vi "ConvertPath.vi"(8 "error in (no error)":errorcluster caption="错误输入（无错误）", 11 "输入路径":path) -> (0 "error out":errorcluster caption="错误输出", 2 "转换后路径":path, 3 "转换前路径":path)   [LabVIEW 2018]
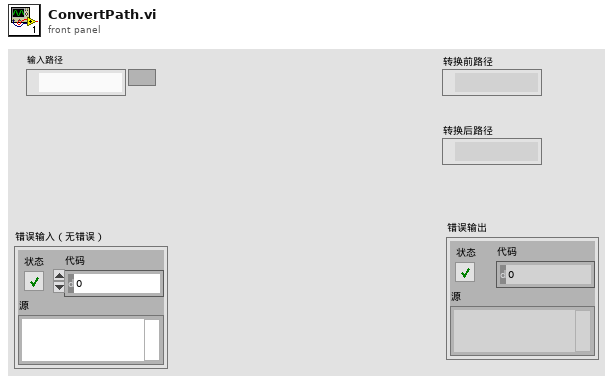
[diagram p1: front panel]
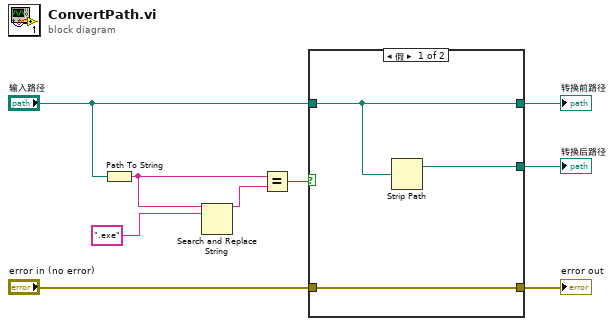
[diagram p0: block diagram]
diagram:
  n1 = Path To String(path="输入路径") -> (string=w7:string)
  n2 = Search and Replace String(input string=w7, search string=".exe") -> (result string=w8:string)  [unwired: 6 in, 3 out]
  n3 = Equal?(x=w7, y=w8) -> (x = y?=w6:bool)
  n4 = case shown="假" w6 {
    tunnel: "输入路径" -> [w12 w13]
    tunnel: [w12 w13] -> w4
    tunnel: [w11 w13] -> w3
    tunnel: "error in (no error)" -> [w10 w14]
    tunnel: [w10 w14] -> w1
    frame False {
      n5 = Strip Path(path=w12) -> (stripped path=w11:path)  [unwired: 1 out]
    }
    frame True {
    }
  }
  "转换后路径" <- w3
  "error out" <- w1
  "转换前路径" <- w4
